vi "Print Sheet ws.vi"(11 "Images":T1[](array[typedef])) -> ()   [LabVIEW 2010]
uses:
  Program Files (x86)/National Instruments/LabVIEW 2010/resource/objmgr/IMAQImage.rc
  <vilib>/vision/Image Controls.llb/IMAQ Image.ctl
panel:
  out "Image 8":T1(plugin-control)
  out "Image 7":T1(plugin-control)
  out "Image 6":T1(plugin-control)
  out "Image 5":T1(plugin-control)
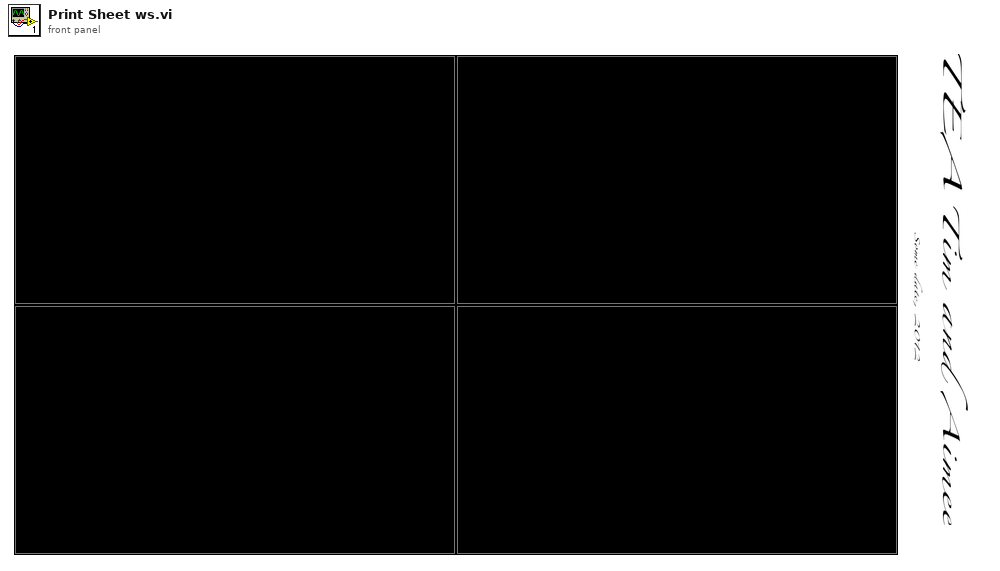
[diagram p1: front panel]
types:
  T1 = typedef "IMAQ Image.ctl" = refnum<image>
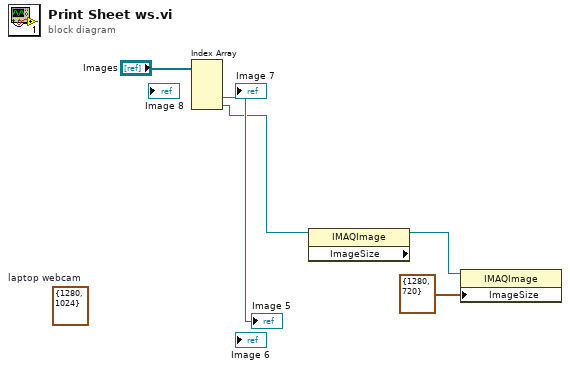
[diagram p0: block diagram]
diagram:
  (unwired) cluster{"x":i32, "y":i32} {"x"=1280, "y"=1024}  # laptop webcam
  n1 = Index Array(array="Images") -> (element #1=w6:T1, element #2=w5:T1, element #3=→"Image 5":T1, element #4=w3:T1)  [unwired: 4 in]
  n2 = property class="IMAQImage"(reference=w3) -> (reference out=w2:T1, "ImageSize"=w1:cluster{"x":i32, "y":i32})  [unwired: 1 in, 1 out]
  n3 = property class="IMAQImage"(reference=w2, "ImageSize"=cluster{"x":i32, "y":i32} {"x"=1280, "y"=720} ("Image Size")) -> (reference out=w7:T1)  [unwired: 1 in, 1 out]
